vi "MesProductDesc.vi"(5 "字段值":string[](array[string]), 7 "字段名":string[](array[string])=["equipment_code", "pallet_code", "location", "product_code", "batch_item", "process_data", "quality_data", "standard", "quality_flag"], 8 "error in":errorcluster, 9 "table":string="collect_board_quality", 10 "connection reference":T1) -> (0 "error out":errorcluster, 2 "connection out":T1, 3 "错误状态":bool)   [LabVIEW 2014]
uses:
  <vilib>/addons/database/Connection.llb/Conn ObjectReference.ctl
  <vilib>/addons/database/Connection.llb/DB Tools Open Connec (String).vi
  <vilib>/addons/database/Connection.llb/Conn Execute.vi
  <vilib>/addons/database/Recordset.llb/Rec Destroy - Connection.vi
  <vilib>/addons/database/NI_Database_API.lvlib
panel:
  out "连接的字符串":string
  # "insert_collect_product_desc"
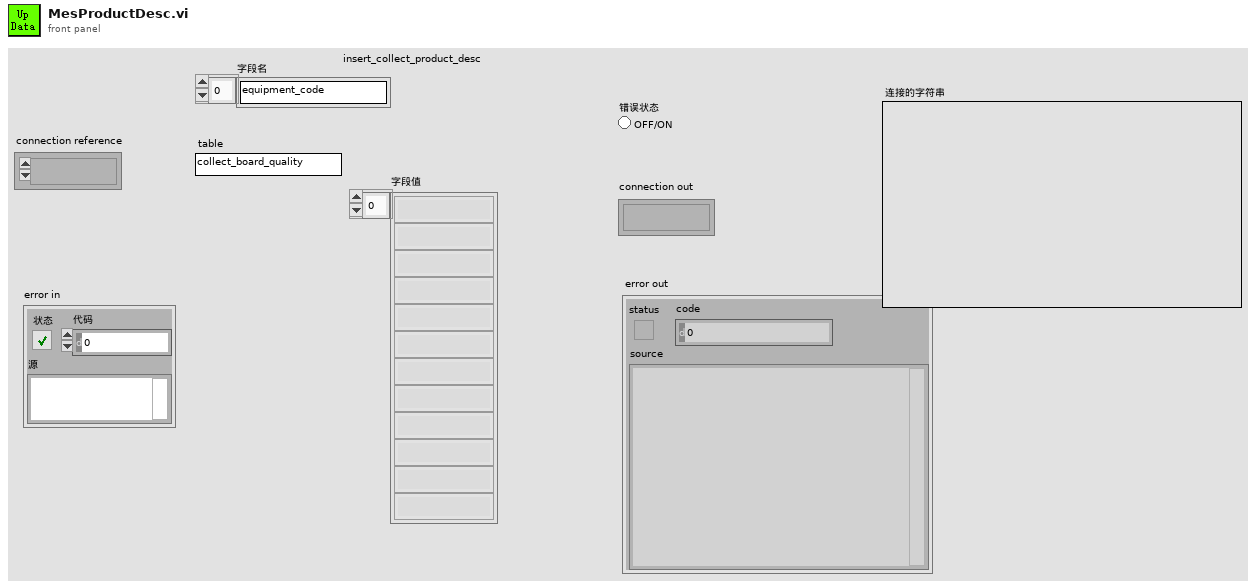
[diagram p1: front panel]
types:
  T1 = typedef "NI_Database_API.lvlib/Conn ObjectReference.ctl" = refnum<k1>
  T2 = typedef "NI_Database_API.lvlib/Rec ObjectReference.ctl" = refnum<k1>
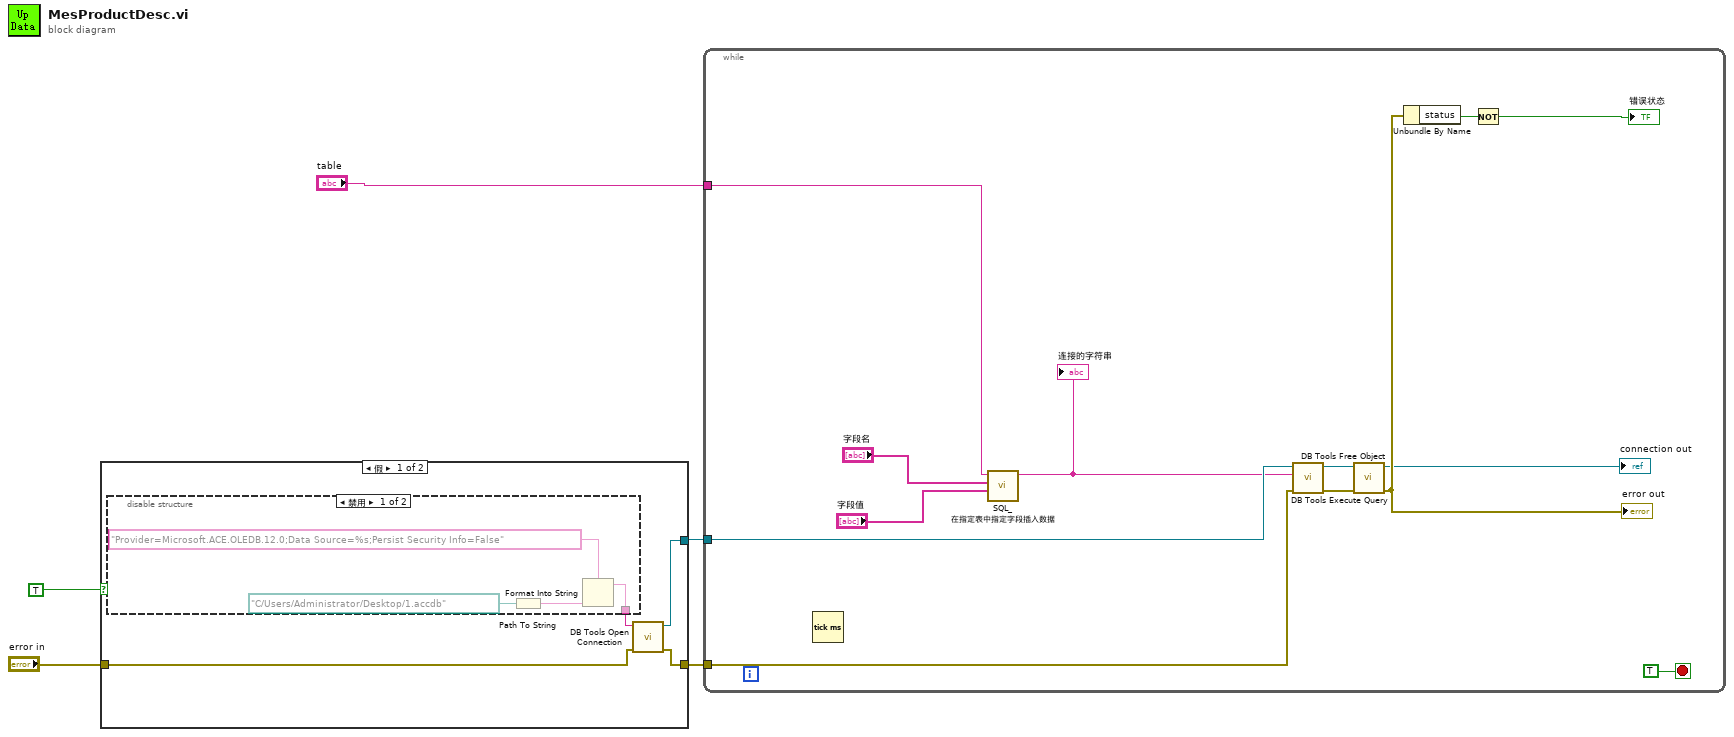
[diagram p0: block diagram]
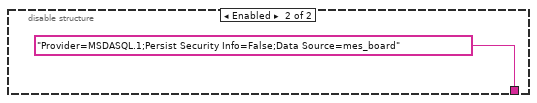
[diagram p2: hidden frame]
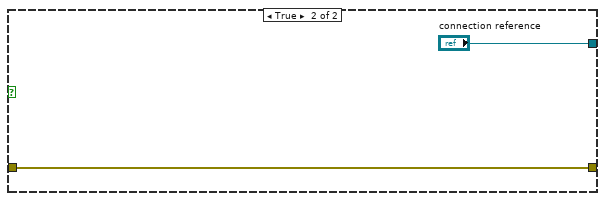
[diagram p3: hidden frame]
diagram:
  n1 = case shown="假" TRUE {
    tunnel: [w9 "connection reference"] -> w3
    tunnel: [w8 w15] -> w4
    tunnel: "error in" -> [w6 w15]
    frame False {
      n2 = disable-structure shown="禁用" {
        disable-tunnel: [w12 "Provider=MSDASQL.1;Persist Security Info=False;Data Source=mes_board" ("connection information")] -> w7
        frame Disabled {
          n3 = Path To String(path=path "C:/Users/Administrator/Desktop/1.accdb" ("路径")) -> (string=w13:string)
          n4 = Format Into String(format string="Provider=Microsoft.ACE.OLEDB.12.0;Data Source=%s;Persist Security Info=False" ("初始字符串"), w13) -> (resulting string=w12:string)  [unwired: 2 in, 1 out]
        }
        frame Enabled {
        }
      }
      n5 = call-poly <vilib>:"DB Tools Open Connection.vi"("error in (no error)"=w6, "connection information"=w7) -> ("error out"=w8:errorcluster, "connection reference"=w9:T1)  [unwired: 6 in]
    }
    frame True {
    }
  }
  n6 = while {
    tunnel: "table" -> [w28]
    tunnel: w3 -> [w27]
    tunnel: w4 -> [w18]
    stop <- TRUE stop-if-true
    n7 = Tick Count (ms)() -> ()  [unwired: 1 out]
    n8 = call "SQL_在指定表中指定字段插入数据.vi"("字段值(字符)"="字段值", "字段名(字符)"="字段名", "表名"=w28) -> ("SQL_在指定表中指定字段插入数据"=w21:string)  [unwired: 7 in, 1 out]
    "连接的字符串" <- w21
    n9 = call-poly <vilib>:"DB Tools Execute Query.vi"("error in (no error)"=w18, "SQL query"=w21, "connection reference"=w27) -> ("error out"=w23:errorcluster, "recordset reference"=w24:T2)  [unwired: 5 in]
    n10 = call-poly <vilib>:"DB Tools Free Object.vi"("error in (no error)"=w23, "recordset reference"=w24) -> ("error out"=w26:errorcluster, "connection reference"=→"connection out":T1)  [unwired: 8 in]
    "error out" <- w26
    n11 = Unbundle By Name(w26) -> ("status"=w22:bool)
    n12 = Not(x=w22) -> (.not. x?=→"错误状态":bool)
  }
